vi "8164B Set WaveLength.vi"(8 "error in":errorcluster, 10 "WaveLength, nm":dbl=1550.0 format="%#_13g", 11 "KeySight 8164B control in":T1) -> (0 "error out":errorcluster, 3 "KeySight 8164B control out":T1)   [LabVIEW 2018, in "KeySight 8164B LAN InstrLib.lvlib"]
uses:
  KeySight 8164B LAN InstrLib.lvlib
  typedefs/KeySight 8164B control.ctl
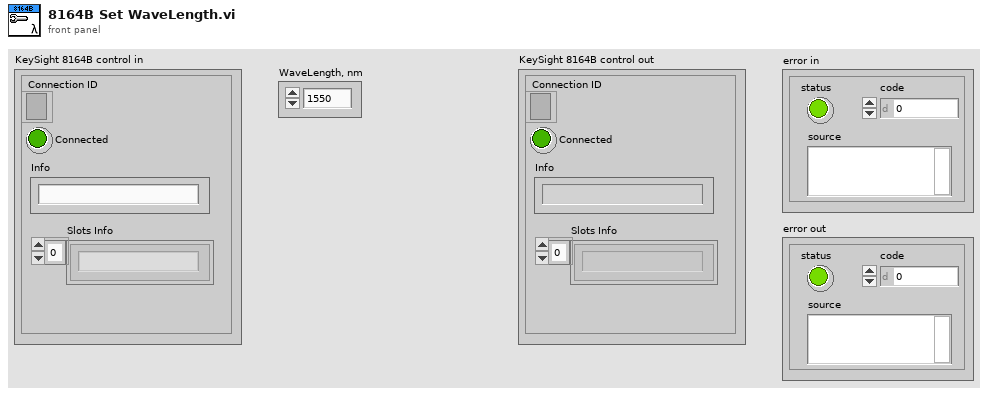
[diagram p1: front panel]
types:
  T1 = typedef "KeySight 8164B LAN InstrLib.lvlib/KeySight 8164B control.ctl" = cluster{"Connection ID":refnum<k5>, "Connected":bool, "Info":string, "Slots Info":string[]}
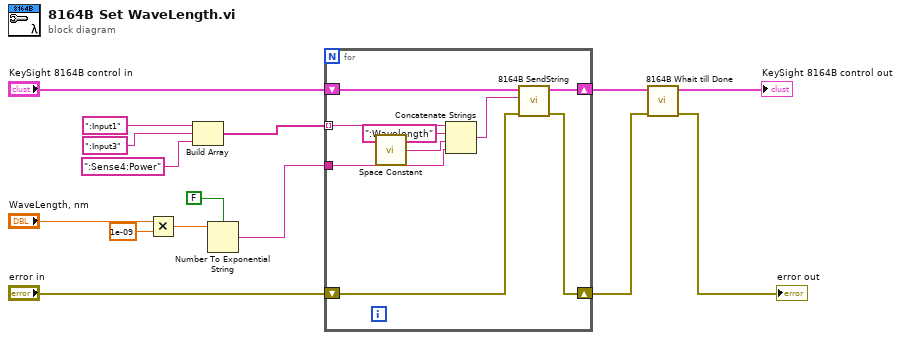
[diagram p0: block diagram]
diagram:
  n1 = Multiply(x="WaveLength, nm", y=1e-09) -> (x*y=w11:dbl)
  n2 = Build Array(":Input1", ":Input3", ":Sense4:Power") -> (w7:string[])
  n3 = Number To Exponential String(number=w11, 1:FALSE ("use system decimal point (T)")) -> (E-format string=w9:string)  [unwired: 2 in]
  n4 = for {
    shift-right: [w23] -> w4
    shift-left: "KeySight 8164B control in" -> [w24]
    shift-right: [w21] -> w3
    shift-left: "error in" -> [w22]
    tunnel: w9 -> [w17]
    tunnel: w7 -> [w20] mode=indexing
    n5 = call <vilib>:"Space Constant.vi"() -> ("String"=w18:string)
    n6 = Concatenate Strings(w20, ":Wavelength" ("string"), w18, w17) -> (w16:string)
    n7 = call "8164B SendString.vi"("error in"=w22, "CMD"=w16, "KeySight 8164B control in"=w24) -> ("error out"=w21:errorcluster, "KeySight 8164B control out"=w23:T1)  [unwired: 7 in]
  }
  n8 = call "8164B Whait till Done.vi"("error in"=w3, "KeySight 8164B control in"=w4) -> ("error out"=→"error out":errorcluster, "KeySight 8164B control out"=→"KeySight 8164B control out":T1)  [unwired: 8 in]
